vi "ACR_APXStand170322.vi"() -> ()   [LabVIEW 2015]
uses:
  <vilib>/Platform/TimedLoop/XDataNode/timing_clust.ctl
  <vilib>/Platform/TimedLoop/XDataNode/nitl_modes.ctl
  <vilib>/Platform/TimedLoop/XDataNode/wakeup.ctl
  <vilib>/Utility/config.llb/Read Key (String).vi
  <userlib>/caLab/Private/Put_DBL-1D_PV-1D.vi
  <vilib>/platform/TimedLoop/XDataNode/XDataNode.xnode
  <vilib>/Platform/TimedLoop/XDataNode/XDNodeRunTimeDep.lvlib
  <vilib>/Utility/config.llb/NI_LVConfig.lvlib
panel:
  out "COM PORT":i32
  in  "AXIS1 spr":bool
  in  "AXIS4 inc":dbl=0.005 min=0.0 max=0.05 step=0.005 format="%.3f"
  in  "AXIS4 spr":bool
  in  "AXIS4 srl":bool
  out "APX:AXIS4_INSPR":dbl
  in  "AXIS2 spr":bool
  in  "AXIS2 srl":bool
  in  "AXIS2 inc":dbl=0.005 min=0.0 max=0.05 step=0.005 format="%.3f"
  out "APX:AXIS2_TRAN":dbl
  in  "AXIS1 srl":bool
  in  "AXIS1 inc":dbl=0.005 min=0.0 max=0.2 step=0.005 format="%.3f"
  out "APX:AXIS1_INSRL":dbl
  in  "APX:AXIS5_ENB":bool
  in  "APX:AXIS4_ENB":bool
  in  "APX:AXIS3_ENB":bool
  in  "APX:AXIS2_ENB":bool
  in  "APX:AXIS1_ENB":bool
  in  "APX:AXIS0_ENB":bool
  out "error out":errorcluster
  out "APX:AXIS5_ENB":bool
  out "APX:AXIS2_EBD":bool
  out "APX:AXIS1_EBD":bool
  out "APX:AXIS3EBD":bool
  out "APX:AXIS4_EBD":bool
  out "APX:AXIS0_EBD":bool
  out "EPICS error out":errorcluster
  out "ACR error out":errorcluster
  in  "stop":bool
  in  "Write String PROG1":string[](array[string])=["detach all", "new all", "clear", "attach master0", "attach slave0 axis0 \"x\"", "axis0 drive on"]
  in  "AXIS5 down":bool
  in  "AXIS5 up":bool
  in  "AXIS5 inc":dbl=0.01 min=0.0 max=0.2 step=0.005 format="%#.6f"
  in  "AXIS3 down":bool
  in  "AXIS3 up":bool
  in  "AXIS3 inc":dbl=0.005 min=0.0 max=0.2 step=0.005 format="%.3f"
  out "APX:AXIS3_SPRSRL":dbl
  in  "AXIS0 inc":dbl=0.005 min=0.0 max=0.2 step=0.005 format="%.3f"
  in  "AXIS0 down":bool
  in  "AXIS0 up":bool
  out "APX:AXIS5_SPRSRL_ACC":dbl
  out "APX:AXIS4_INSPR_ACC":dbl
  out "APX:AXIS3_SPRSRL_ACC":dbl
  out "APX:AXIS2_TRAN_ACC":dbl
  out "APX:AXIS1_INSRL_ACC":dbl
  out "APX:AXIS0 ZSRL_ACC":dbl
  out "APX:AXIS5_SPRSRL_VEL":dbl
  out "APX:AXIS4_INSPR_VEL":dbl
  out "APX:AXIS3_SPRSRL_VEL":dbl
  out "APX:AXIS2_TRAN_VEL":dbl
  out "APX:AXIS1_INSRL_VEL":dbl
  out "APX:AXIS0_ZSRL_VEL":dbl
  out "APX:AXIS5_SPRSRL":dbl
  in  "nPort":i32=28
  in  "Sampling Time (s)":dbl=0.2
  out "APX:AXIS0_ZSRL":dbl
  in  "Read error in \n(no error)":errorcluster
  in  "Move CMD":string="x/100"
  in  "OK Button":bool
  in  "Write String PROG0":string[](array[string])=["detach all", "new all", "clear", "attach master0", "attach slave0 axis0 \"x\"", "axis0 drive on"]
  out "Terminal Status":bool
  in  "ComACRServerLib.IChannel":refnum<k7>
  in  "bstrIP Property":string="192.168.10.40"
  out "Connect error out":errorcluster
  in  "Connect error in \n(no error)":errorcluster
  # "Ethernet Configuration"
  # "Command"
  # "Configure"
  # "APX\nACR9000 USB"
  # "detach all\nnew all\nclear\nattach master0\nattach slave0 axis0 \"x\"\naxis0 drive on"
  # "Position"
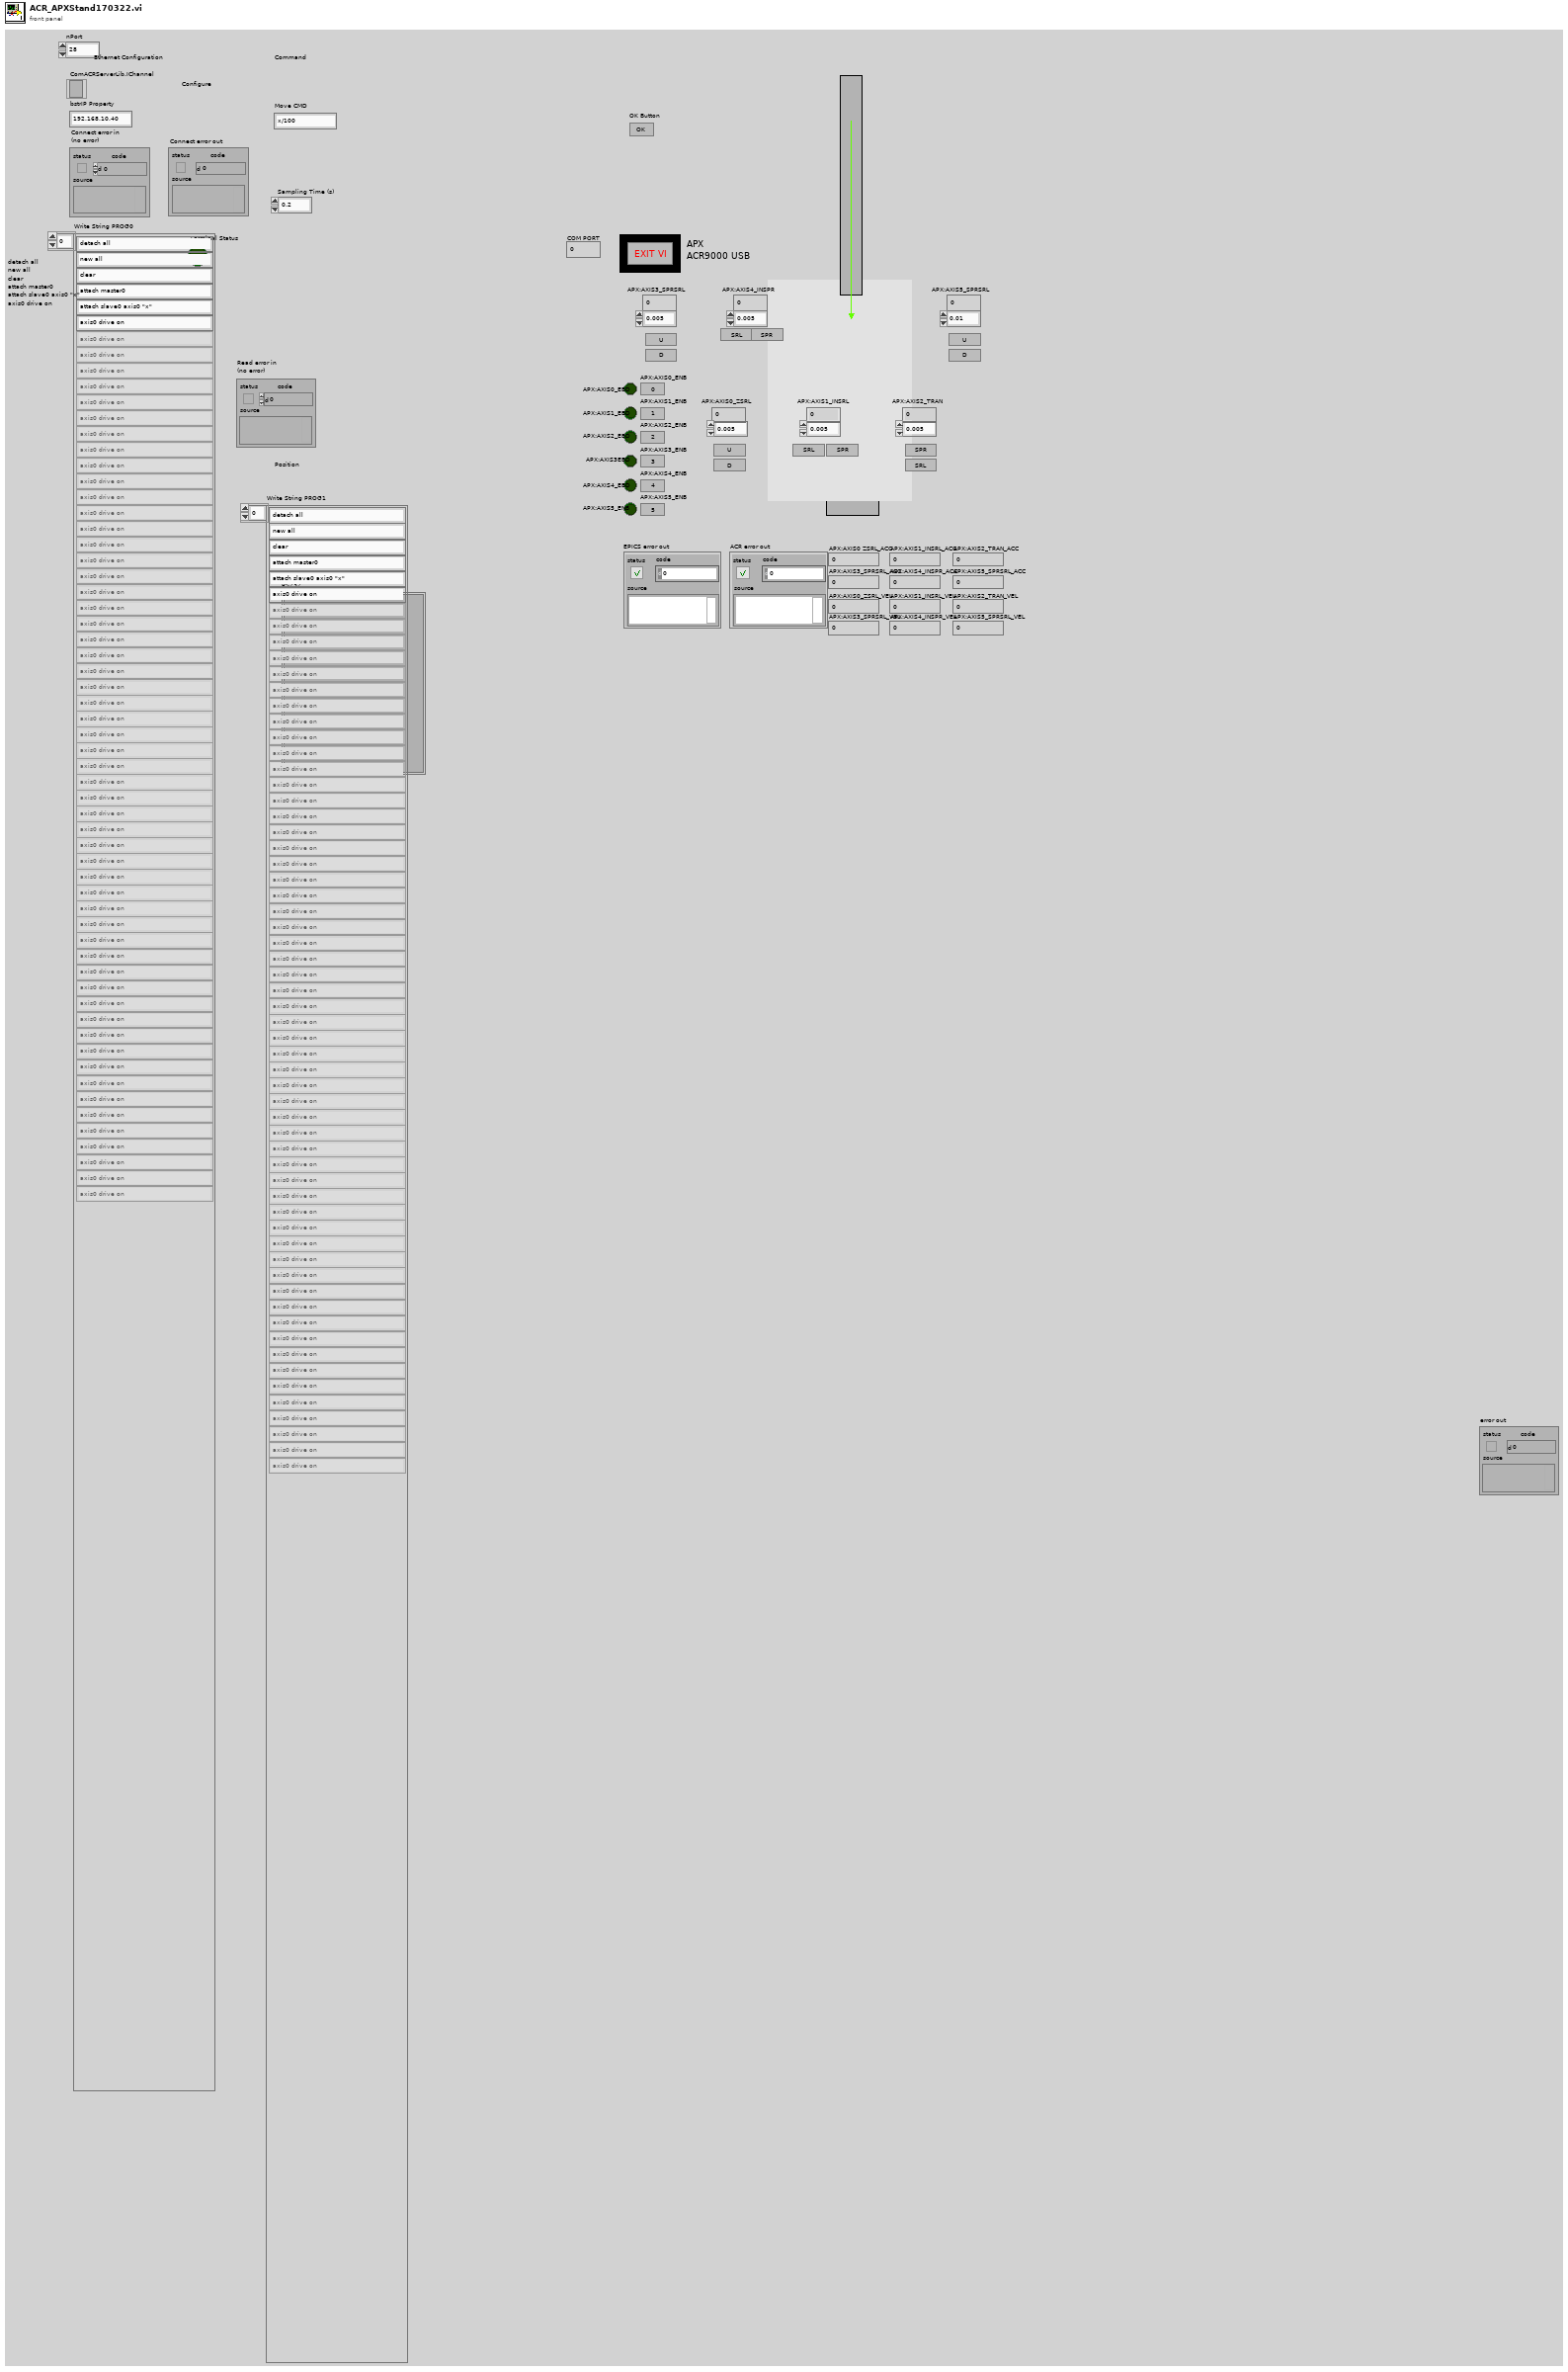
[diagram p1: front panel]
types:
  T1 = typedef "NI_LVConfig.lvlib/Config Data RefNum.ctl" = refnum<k1>
  T2 = typedef "XDNodeRunTimeDep.lvlib/timing_clust.ctl" = cluster{"Expected End [f-1]":u64, "Actual End [f-1]":u64, "Finished Late? [f-1]":bool, "Expected End [i-1]":u64, "Actual End [i-1]":u64, "Finished Late? [i-1]":bool, "Expected Start [i]":u64, "Actual Start [i]":u64, "Expected Start [f]":u64, "Actual Start [f]":u64, "Source Name":string, "Structure Name":string, "Period":i64, "Deadline":i64, "Offset":i64, "Start":i64, "Priority":i32, "Timeout":i32, "Mode":T3, "Wakeup Reason":T4, "Error":errorcluster, "Source Type":string, "Secondary Source Type":string, "Global End Time":u64, "Global Start Time":u64, "Frame Duration":u64, "Iteration Duration":u64, "Assigned CPU":i32, "I/O Scan Engine Mode":u32}
  T3 = typedef "XDNodeRunTimeDep.lvlib/nitl_modes.ctl" = enum32{"No Change", "Process missed periods, maintain original phase", "Discard missed periods, maintain original phase", "Process missed periods, ignore original phase", "Discard missed periods, ignore original phase"}
  T4 = typedef "XDNodeRunTimeDep.lvlib/wakeup.ctl" = enum32{"Normal", "Aborted", "Asynchronous wakeup", "Timing source error", "Timed loop error", "Timeout"}
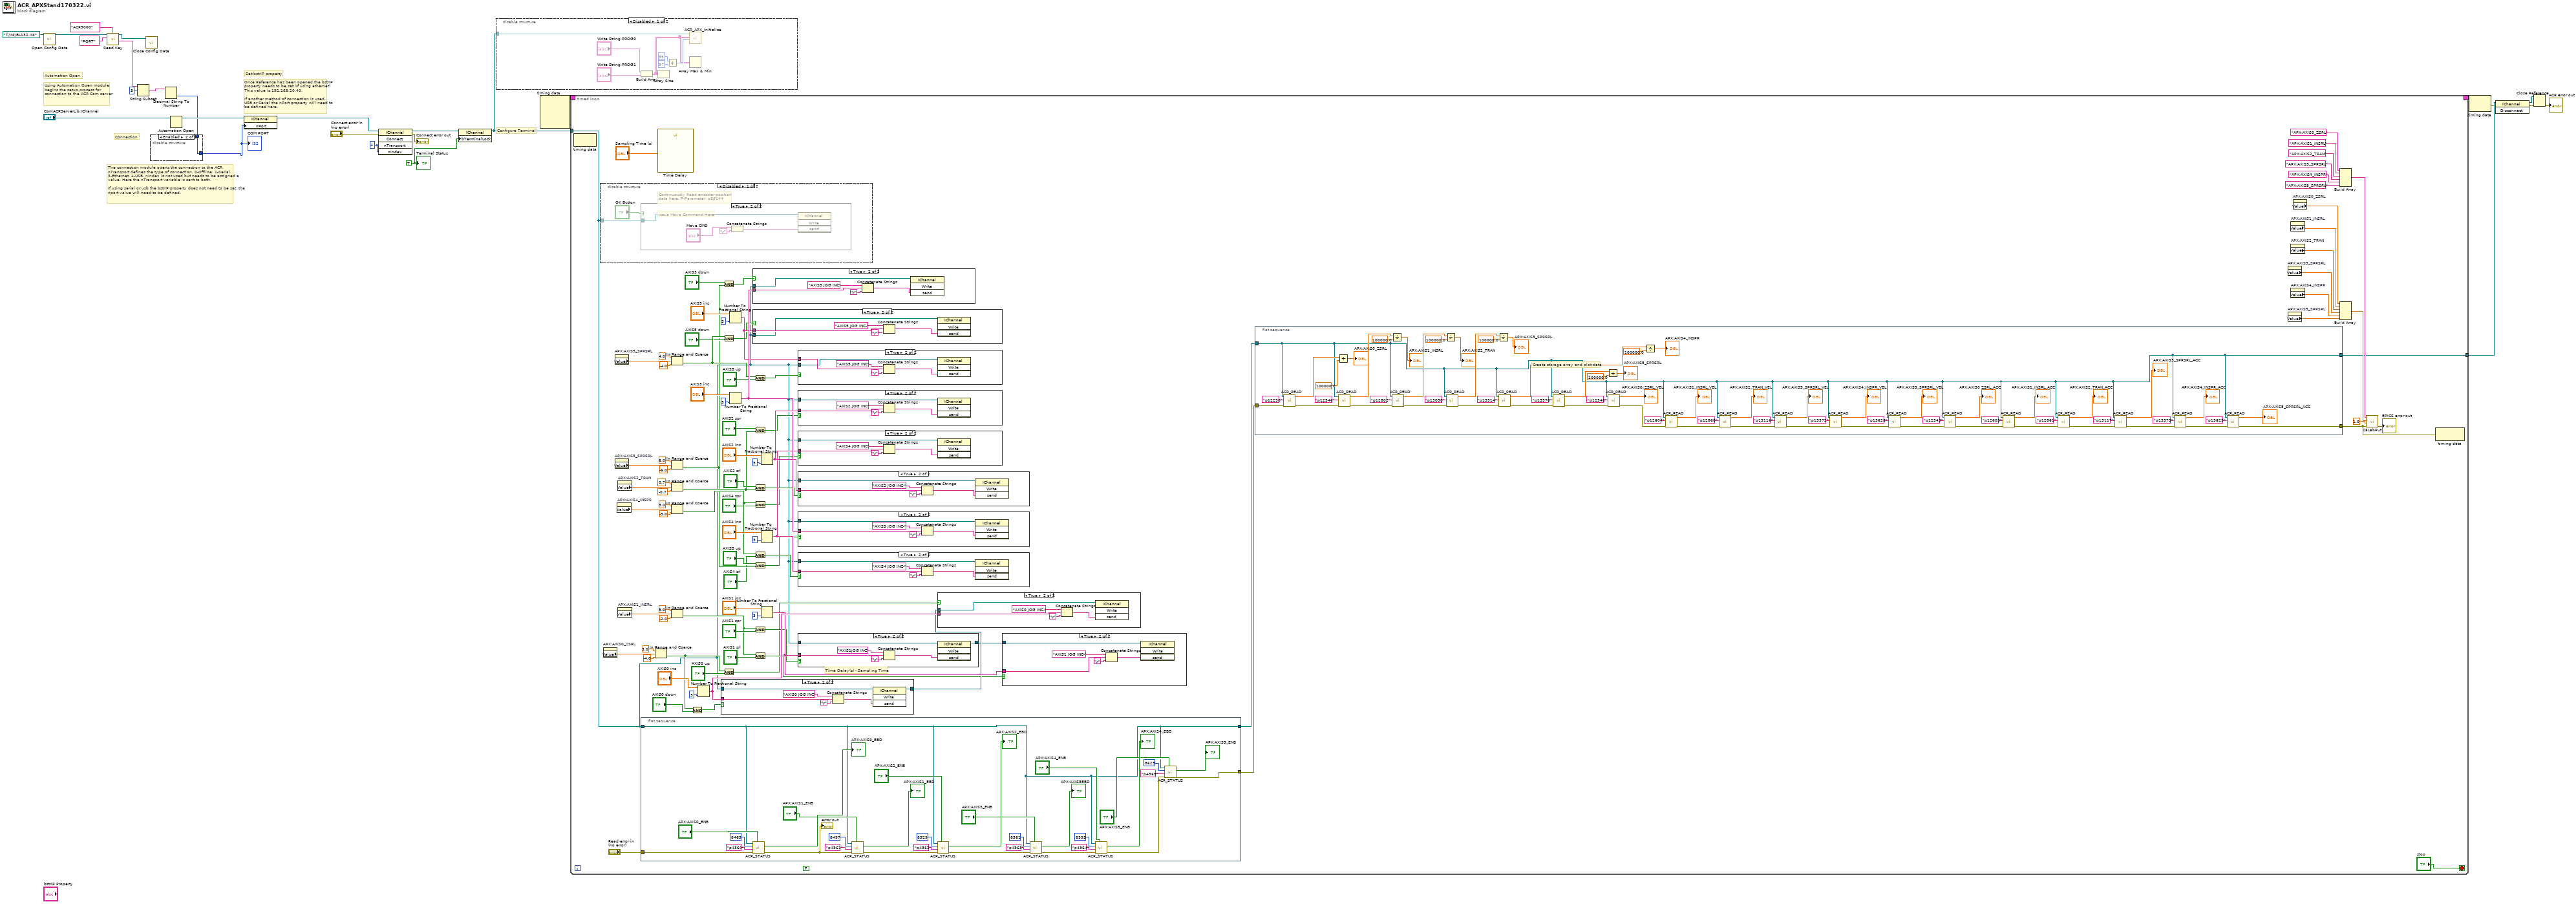
[diagram p0: block diagram]
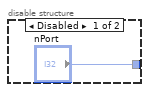
[diagram p2: hidden frame]
diagram:
  w19 = TRUE
  w23 = 4
  # "Configure Terminal"
  # "Using Automation Open module begins the setup process for connection to the ACR Com server"
  # "Automation Open"
  # "Once Reference has been opened,the bstrIP property needs to be set.(If using ethernet) This value is 192.168.10.40. \n\nIf another method of connection is used, USB or Serial the nPort property will need to be defined here."
  # "Set bstrIP property"
  # "The connection module opens the connection to the ACR. nTransport defines the type of connection. 0-Offline, 2-Serial, 3-Ethernet, 4-USB. nIndex is not used but needs to be assigned a value. Here the nTransport variable is sent to both.\n\nIf using serial or usb the bstrIP property does not need to be set; the nport value will need to be defined."
  # "Connection"
  n1 = call <vilib>:"Open Config Data.vi"("configuration file path"=path "T:/INI/BL132.INI") -> ("refnum"=w7:T1)  [unwired: 8 in, 2 out]
  n2 = call-poly <vilib>:"Read Key.vi"("section"="ACR9000" ("y"), "key"="PORT" ("y"), "refnum"=w7) -> ("value"=w5:string, "refnum out"=w6:T1)  [unwired: 5 in, 2 out]
  n3 = String Subset(string=w5, offset (0)=3) -> (substring=w3:string)  [unwired: 1 in]
  n4 = call <vilib>:"Close Config Data.vi"("refnum"=w6) -> ()  [unwired: 9 in, 2 out]
  n5 = Decimal String To Number(string=w3) -> (number=w1:i32)  [unwired: 2 in, 1 out]
  n6 = disable-structure shown="Enabled" {
    disable-tunnel: ["nPort" w28] -> w2
    disable-tunnel: w1 -> [_ w28]
    frame Disabled {
    }
    frame Enabled {
    }
  }
  "COM PORT" <- w2
  n7 = Automation Open(Automation Refnum="ComACRServerLib.IChannel") -> (Automation Refnum=w22:refnum<k7>)  [unwired: 1 in, 3 out]
  n8 = property class="IChannel"(reference=w22, "nPort"=w2) -> (reference out=w21:refnum<k7>)  [unwired: 1 in, 1 out]
  n9 = invoke class="IChannel" method="Connect"(reference=w21, error in="Connect error in \n(no error)", "nTransport"=w23, "nIndex"=w23) -> (reference out=w20:refnum<k7>, error out=→"Connect error out":errorcluster)  [unwired: 1 in, 3 out]
  n10 = property class="IChannel"(reference=w20, "bTerminalLock"=w19) -> (reference out=w18:refnum<k7>)  [unwired: 1 in, 1 out]
  n11 = disable-structure shown="Disabled" {
    disable-tunnel: w18 -> [w35 _]
    frame Disabled {
      n12 = Build Array("Write String PROG0", "Write String PROG1") -> (w29:string[][])
      n13 = Array Size(array=w29) -> ()  [unwired: 1 out]
      n14 = Add(x=99, y=97) -> (x+y=w32:i32)
      n15 = call "ACR_APX_Initialize.vi"("Numeric"=w32, "Array"=w29, "Automation Refnum in"=w35) -> ()  [unwired: 9 in]
      n16 = Array Max & Min(array=w29) -> ()  [unwired: 4 out]
    }
    frame Enabled {
    }
  }
  n17 = node-c288() -> (w17:T2)  [unwired: 4 in]
  n18 = timed-loop {
    tunnel: w18 -> [w40]
    timing: w17 -> [_]
    timing-out: [_] -> w16
    tunnel: [w36] -> w13
    stop <- "stop" stop-if-true
    (unwired) FALSE
    # "Time Delay(s) - Sampling Time"
    n19 = node-c288() -> ()  [unwired: 1 in, 1 out]
    n20 = disable-structure shown="Disabled" {
      disable-tunnel: w40 -> [w228 _]
      frame Disabled {
        # "Continuously Read encoder position\ndata here. P-Parameter: p38144"
        n21 = case shown="True" "OK Button" {
          tunnel: w228 -> [_ w230]
          frame False {
          }
          frame True {
            # "Issue Move Command Here"
            n22 = Concatenate Strings("Move CMD", "\r") -> (w233:string)
            n23 = invoke class="IChannel" method="Write"(reference=w230, "send"=w233) -> ()  [unwired: 2 in, 4 out]
          }
        }
      }
      frame Enabled {
      }
    }
    n24 = property on="APX:AXIS0_ZSRL" class="DigNum (strict)"() -> ("Value"=w48:dbl)  [unwired: 2 in, 2 out]
    n25 = property on="APX:AXIS5_SPRSRL" class="DigNum (strict)"() -> ("Value"=w90:dbl)  [unwired: 2 in, 2 out]
    n26 = property on="APX:AXIS3_SPRSRL" class="DigNum (strict)"() -> ("Value"=w74:dbl)  [unwired: 2 in, 2 out]
    n27 = property on="APX:AXIS4_INSPR" class="DigNum (strict)"() -> ("Value"=w66:dbl)  [unwired: 2 in, 2 out]
    n28 = property on="APX:AXIS2_TRAN" class="DigNum (strict)"() -> ("Value"=w82:dbl)  [unwired: 2 in, 2 out]
    n29 = property on="APX:AXIS1_INSRL" class="DigNum (strict)"() -> ("Value"=w56:dbl)  [unwired: 2 in, 2 out]
    n30 = flat-sequence {
      tunnel: "Read error in \n(no error)" -> [w227]
      tunnel: [w196] -> w37
      tunnel: w40 -> [w196]
      tunnel: [w198] -> w38
      frame #0 {
        n31 = call "ACR_STATUS.vi"("EnableDrive"="APX:AXIS0_ENB", "error in (no error)"=w227, "bstrRequest"="p4360", "nBit"=8465, "Automation Refnum in"=w196) -> ("error out"=w222:errorcluster, "DrvEnaOut"=→"APX:AXIS0_EBD":bool)  [unwired: 4 in, 1 out]
        "error out" <- w222
        n32 = call "ACR_STATUS.vi"("EnableDrive"="APX:AXIS1_ENB", "error in (no error)"=w222, "bstrRequest"="p4361", "nBit"=8497, "Automation Refnum in"=w196) -> ("error out"=w217:errorcluster, "DrvEnaOut"=→"APX:AXIS1_EBD":bool)  [unwired: 4 in, 1 out]
        n33 = call "ACR_STATUS.vi"("EnableDrive"="APX:AXIS2_ENB", "error in (no error)"=w217, "bstrRequest"="p4362", "nBit"=8529, "Automation Refnum in"=w196) -> ("error out"=w212:errorcluster, "DrvEnaOut"=→"APX:AXIS2_EBD":bool)  [unwired: 4 in, 1 out]
        n34 = call "ACR_STATUS.vi"("EnableDrive"="APX:AXIS3_ENB", "error in (no error)"=w212, "bstrRequest"="p4363", "nBit"=8561, "Automation Refnum in"=w196) -> ("error out"=w207:errorcluster, "DrvEnaOut"=→"APX:AXIS3EBD":bool)  [unwired: 4 in, 1 out]
        n35 = call "ACR_STATUS.vi"("EnableDrive"="APX:AXIS4_ENB", "error in (no error)"=w207, "bstrRequest"="p4364", "nBit"=8593, "Automation Refnum in"=w196) -> ("error out"=w202:errorcluster, "DrvEnaOut"=→"APX:AXIS4_EBD":bool)  [unwired: 4 in, 1 out]
        n36 = call "ACR_STATUS.vi"("EnableDrive"="APX:AXIS5_ENB", "error in (no error)"=w202, "bstrRequest"="p4365", "nBit"=8625, "Automation Refnum in"=w196) -> ("error out"=w198:errorcluster, "DrvEnaOut"=→"APX:AXIS5_ENB":bool)  [unwired: 4 in, 1 out]
      }
    }
    n37 = In Range and Coerce(upper limit=5.0, x=w48, lower limit=-4.0) -> (In Range?=w43:bool)  [unwired: 1 out]
    n38 = call "Time Delay"("Delay Time (s)"="Sampling Time (s)") -> ()  [unwired: 1 in, 10 out]
    n39 = In Range and Coerce(upper limit=4.0, x=w90, lower limit=-4.0) -> (In Range?=w85:bool)  [unwired: 1 out]
    n40 = In Range and Coerce(upper limit=6.0, x=w74, lower limit=-6.0) -> (In Range?=w71:bool)  [unwired: 1 out]
    n41 = In Range and Coerce(upper limit=0.7, x=w82, lower limit=-0.7) -> (In Range?=w79:bool)  [unwired: 1 out]
    n42 = In Range and Coerce(upper limit=3.0, x=w66, lower limit=-3.0) -> (In Range?=w64:bool)  [unwired: 1 out]
    n43 = In Range and Coerce(upper limit=3.0, x=w56, lower limit=-2.0) -> (In Range?=w51:bool)  [unwired: 1 out]
    n44 = And(x=w43, y="AXIS0 down") -> (x .and. y?=w46:bool)
    n45 = Number To Fractional String(number="AXIS0 inc", precision (6)=i16 3) -> (F-format string=w124:string)  [unwired: 2 in]
    n46 = case shown="True" w46 {
      tunnel: w124 -> [_ w295]
      tunnel: w40 -> [w290 w292]
      tunnel: [w290 w291] -> w108
      frame False {
      }
      frame True {
        n47 = Concatenate Strings("AXIS0 JOG INC", w295, "\r") -> (w293:string)
        n48 = invoke class="IChannel" method="Write"(reference=w292, "send"=w293) -> (reference out=w291:refnum<k7>)  [unwired: 2 in, 3 out]
      }
    }
    n49 = And(x="AXIS3 down", y=w71) -> (x .and. y?=w68:bool)
    n50 = And(x=w85, y="AXIS5 down") -> (x .and. y?=w83:bool)
    n51 = And(x=w43, y="AXIS0 up") -> (x .and. y?=w44:bool)
    n52 = Number To Fractional String(number="AXIS5 inc", precision (6)=i16 3) -> (F-format string=w110:string)  [unwired: 2 in]
    n53 = Number To Fractional String(number="AXIS3 inc", precision (6)=i16 3) -> (F-format string=w116:string)  [unwired: 2 in]
    n54 = case shown="True" w68 {
      tunnel: w116 -> [_ w261]
      tunnel: w40 -> [_ w258]
      frame False {
      }
      frame True {
        n55 = Concatenate Strings("AXIS3 JOG INC", w261, "\r") -> (w259:string)
        n56 = invoke class="IChannel" method="Write"(reference=w258, "send"=w259) -> ()  [unwired: 2 in, 4 out]
      }
    }
    n57 = case shown="True" w83 {
      tunnel: w110 -> [_ w246]
      tunnel: w40 -> [_ w243]
      frame False {
      }
      frame True {
        n58 = Concatenate Strings("AXIS5 JOG INC-", w246, "\r") -> (w244:string)
        n59 = invoke class="IChannel" method="Write"(reference=w243, "send"=w244) -> ()  [unwired: 2 in, 4 out]
      }
    }
    n60 = And(x=w85, y="AXIS5 up") -> (x .and. y?=w86:bool)
    n61 = And(x="AXIS2 spr", y=w79) -> (x .and. y?=w75:bool)
    n62 = And(x="AXIS2 srl", y=w79) -> (x .and. y?=w77:bool)
    n63 = And(x=w64, y="AXIS4 spr") -> (x .and. y?=w62:bool)
    n64 = And(x=w64, y="AXIS4 srl") -> (x .and. y?=w60:bool)
    n65 = And(x="AXIS3 up", y=w71) -> (x .and. y?=w67:bool)
    n66 = And(x=w51, y="AXIS1 spr") -> (x .and. y?=w52:bool)
    n67 = And(x=w51, y="AXIS1 srl") -> (x .and. y?=w54:bool)
    n68 = Number To Fractional String(number="AXIS2 inc", precision (6)=i16 3) -> (F-format string=w119:string)  [unwired: 2 in]
    n69 = Number To Fractional String(number="AXIS4 inc", precision (6)=i16 3) -> (F-format string=w113:string)  [unwired: 2 in]
    n70 = Number To Fractional String(number="AXIS1 inc", precision (6)=i16 3) -> (F-format string=w122:string)  [unwired: 2 in]
    n71 = case shown="True" w86 {
      tunnel: w110 -> [_ w241]
      tunnel: w40 -> [_ w238]
      frame False {
      }
      frame True {
        n72 = Concatenate Strings("AXIS5 JOG INC", w241, "\r") -> (w239:string)
        n73 = invoke class="IChannel" method="Write"(reference=w238, "send"=w239) -> ()  [unwired: 2 in, 4 out]
      }
    }
    n74 = case shown="True" w75 {
      tunnel: w119 -> [_ w271]
      tunnel: w40 -> [_ w268]
      frame False {
      }
      frame True {
        n75 = Concatenate Strings("AXIS2 JOG INC", w271, "\r") -> (w269:string)
        n76 = invoke class="IChannel" method="Write"(reference=w268, "send"=w269) -> ()  [unwired: 2 in, 4 out]
      }
    }
    n77 = case shown="True" w62 {
      tunnel: w113 -> [_ w251]
      tunnel: w40 -> [_ w248]
      frame False {
      }
      frame True {
        n78 = Concatenate Strings("AXIS4 JOG INC", w251, "\r") -> (w249:string)
        n79 = invoke class="IChannel" method="Write"(reference=w248, "send"=w249) -> ()  [unwired: 2 in, 4 out]
      }
    }
    n80 = case shown="True" w77 {
      tunnel: w119 -> [_ w276]
      tunnel: w40 -> [_ w274]
      frame False {
      }
      frame True {
        n81 = Concatenate Strings("AXIS2 JOG INC-", w276, "\r") -> (w273:string)
        n82 = invoke class="IChannel" method="Write"(reference=w274, "send"=w273) -> ()  [unwired: 2 in, 4 out]
      }
    }
    n83 = case shown="True" w67 {
      tunnel: w116 -> [_ w266]
      tunnel: w40 -> [_ w263]
      frame False {
      }
      frame True {
        n84 = Concatenate Strings("AXIS3 JOG INC-", w266, "\r") -> (w264:string)
        n85 = invoke class="IChannel" method="Write"(reference=w263, "send"=w264) -> ()  [unwired: 2 in, 4 out]
      }
    }
    n86 = case shown="True" w60 {
      tunnel: w113 -> [_ w256]
      tunnel: w40 -> [_ w253]
      frame False {
      }
      frame True {
        n87 = Concatenate Strings("AXIS4 JOG INC-", w256, "\r") -> (w254:string)
        n88 = invoke class="IChannel" method="Write"(reference=w253, "send"=w254) -> ()  [unwired: 2 in, 4 out]
      }
    }
    n89 = case shown="True" w52 {
      tunnel: w122 -> [_ w283]
      tunnel: w40 -> [w278 w280]
      tunnel: [w278 w279] -> w107
      frame False {
      }
      frame True {
        n90 = Concatenate Strings("AXIS1JOG INC", w283, "\r") -> (w281:string)
        n91 = invoke class="IChannel" method="Write"(reference=w280, "send"=w281) -> (reference out=w279:refnum<k7>)  [unwired: 2 in, 3 out]
      }
    }
    n92 = case shown="True" w44 {
      tunnel: w124 -> [_ w300]
      tunnel: w108 -> [_ w297]
      frame False {
      }
      frame True {
        n93 = Concatenate Strings("AXIS0 JOG INC-", w300, "\r") -> (w298:string)
        n94 = invoke class="IChannel" method="Write"(reference=w297, "send"=w298) -> ()  [unwired: 2 in, 4 out]
      }
    }
    n95 = case shown="True" w54 {
      tunnel: w122 -> [_ w288]
      tunnel: w107 -> [_ w285]
      frame False {
      }
      frame True {
        n96 = Concatenate Strings("AXIS1 JOG INC-", w288, "\r") -> (w286:string)
        n97 = invoke class="IChannel" method="Write"(reference=w285, "send"=w286) -> ()  [unwired: 2 in, 4 out]
      }
    }
    n98 = flat-sequence {
      tunnel: [w130] -> w42
      tunnel: w38 -> [w129]
      tunnel: w37 -> [w128]
      tunnel: [w128] -> w36
      frame #0 {
        # "Create storage array and plot data"
        n99 = call "ACR_READ.vi"("error in (no error)"=w129, "Actual"="p12290", "Automation Refnum in"=w128) -> ("error out"=w194:errorcluster, "AXIS0"=w147:dbl)  [unwired: 7 in]
        n100 = Divide(x=w147, y=100000.0) -> (x/y=→"APX:AXIS0_ZSRL":dbl)
        n101 = call "ACR_READ.vi"("error in (no error)"=w194, "Actual"="p12546", "Automation Refnum in"=w128) -> ("error out"=w193:errorcluster, "AXIS0"=w144:dbl)  [unwired: 7 in]
        n102 = Divide(x=w144, y=100000.0) -> (x/y=→"APX:AXIS1_INSRL":dbl)
        n103 = call "ACR_READ.vi"("error in (no error)"=w193, "Actual"="p12802", "Automation Refnum in"=w128) -> ("error out"=w192:errorcluster, "AXIS0"=w141:dbl)  [unwired: 7 in]
        n104 = Divide(x=w141, y=100000.0) -> (x/y=→"APX:AXIS2_TRAN":dbl)
        n105 = call "ACR_READ.vi"("error in (no error)"=w192, "Actual"="p13058", "Automation Refnum in"=w128) -> ("error out"=w191:errorcluster, "AXIS0"=w138:dbl)  [unwired: 7 in]
        n106 = Divide(x=w138, y=100000.0) -> (x/y=→"APX:AXIS3_SPRSRL":dbl)
        n107 = call "ACR_READ.vi"("error in (no error)"=w191, "Actual"="p13314", "Automation Refnum in"=w128) -> ("error out"=w190:errorcluster, "AXIS0"=w135:dbl)  [unwired: 7 in]
        n108 = call "ACR_READ.vi"("error in (no error)"=w190, "Actual"="p13570", "Automation Refnum in"=w128) -> ("error out"=w179:errorcluster, "AXIS0"=w132:dbl)  [unwired: 7 in]
        n109 = Divide(x=w132, y=100000.0) -> (x/y=→"APX:AXIS5_SPRSRL":dbl)
        n110 = call "ACR_READ.vi"("error in (no error)"=w179, "Actual"="p12348", "Automation Refnum in"=w128) -> ("error out"=w184:errorcluster, "AXIS0"=→"APX:AXIS0_ZSRL_VEL":dbl)  [unwired: 7 in]
        n111 = Divide(x=w135, y=100000.0) -> (x/y=→"APX:AXIS4_INSPR":dbl)
        n112 = call "ACR_READ.vi"("error in (no error)"=w184, "Actual"="p12604", "Automation Refnum in"=w128) -> ("error out"=w183:errorcluster, "AXIS0"=→"APX:AXIS1_INSRL_VEL":dbl)  [unwired: 7 in]
        n113 = call "ACR_READ.vi"("error in (no error)"=w183, "Actual"="p12860", "Automation Refnum in"=w128) -> ("error out"=w182:errorcluster, "AXIS0"=→"APX:AXIS2_TRAN_VEL":dbl)  [unwired: 7 in]
        n114 = call "ACR_READ.vi"("error in (no error)"=w182, "Actual"="p13116", "Automation Refnum in"=w128) -> ("error out"=w181:errorcluster, "AXIS0"=→"APX:AXIS3_SPRSRL_VEL":dbl)  [unwired: 7 in]
        n115 = call "ACR_READ.vi"("error in (no error)"=w181, "Actual"="p13372", "Automation Refnum in"=w128) -> ("error out"=w180:errorcluster, "AXIS0"=→"APX:AXIS4_INSPR_VEL":dbl)  [unwired: 7 in]
        n116 = call "ACR_READ.vi"("error in (no error)"=w180, "Actual"="p13628", "Automation Refnum in"=w128) -> ("error out"=w155:errorcluster, "AXIS0"=→"APX:AXIS5_SPRSRL_VEL":dbl)  [unwired: 7 in]
        n117 = call "ACR_READ.vi"("error in (no error)"=w155, "Actual"="p12349", "Automation Refnum in"=w128) -> ("error out"=w166:errorcluster, "AXIS0"=→"APX:AXIS0 ZSRL_ACC":dbl)  [unwired: 7 in]
        n118 = call "ACR_READ.vi"("error in (no error)"=w166, "Actual"="p12605", "Automation Refnum in"=w128) -> ("error out"=w165:errorcluster, "AXIS0"=→"APX:AXIS1_INSRL_ACC":dbl)  [unwired: 7 in]
        n119 = call "ACR_READ.vi"("error in (no error)"=w165, "Actual"="p12861", "Automation Refnum in"=w128) -> ("error out"=w164:errorcluster, "AXIS0"=→"APX:AXIS2_TRAN_ACC":dbl)  [unwired: 7 in]
        n120 = call "ACR_READ.vi"("error in (no error)"=w164, "Actual"="p13117", "Automation Refnum in"=w128) -> ("error out"=w163:errorcluster, "AXIS0"=→"APX:AXIS3_SPRSRL_ACC":dbl)  [unwired: 7 in]
        n121 = call "ACR_READ.vi"("error in (no error)"=w163, "Actual"="p13373", "Automation Refnum in"=w128) -> ("error out"=w162:errorcluster, "AXIS0"=→"APX:AXIS4_INSPR_ACC":dbl)  [unwired: 7 in]
        n122 = call "ACR_READ.vi"("error in (no error)"=w162, "Actual"="p13629", "Automation Refnum in"=w128) -> ("error out"=w130:errorcluster, "AXIS0"=→"APX:AXIS5_SPRSRL_ACC":dbl)  [unwired: 7 in]
      }
    }
    n123 = property on="APX:AXIS3_SPRSRL" class="DigNum (strict)"() -> ("Value"=w95:dbl)  [unwired: 2 in, 2 out]
    n124 = property on="APX:AXIS5_SPRSRL" class="DigNum (strict)"() -> ("Value"=w93:dbl)  [unwired: 2 in, 2 out]
    n125 = property on="APX:AXIS1_INSRL" class="DigNum (strict)"() -> ("Value"=w97:dbl)  [unwired: 2 in, 2 out]
    n126 = property on="APX:AXIS2_TRAN" class="DigNum (strict)"() -> ("Value"=w96:dbl)  [unwired: 2 in, 2 out]
    n127 = property on="APX:AXIS4_INSPR" class="DigNum (strict)"() -> ("Value"=w94:dbl)  [unwired: 2 in, 2 out]
    n128 = property on="APX:AXIS0_ZSRL" class="DigNum (strict)"() -> ("Value"=w98:dbl)  [unwired: 2 in, 2 out]
    n129 = Build Array("APX:AXIS0_ZSRL", "APX:AXIS1_INSRL", "APX:AXIS2_TRAN", "APX:AXIS3_SPRSRL", "APX:AXIS4_INSPR", "APX:AXIS5_SPRSRL") -> (w91:string[])
    n130 = Build Array(w98, w97, w96, w95, w94, w93) -> (w92:dbl[])
    n131 = call-poly <userlib>:"CaLabPut.vi"("Error in (no error)"=w42, "Timeout (3)"=1.0, "Values"=w92, "PV Names"=w91) -> ("Error out"=→"EPICS error out":errorcluster)  [unwired: 4 in, 3 out]
    n132 = node-c288(w42) -> ()  [unwired: 1 out]
  }
  n133 = node-c288(w16) -> (w11:errorcluster)
  n134 = invoke class="IChannel" method="Disconnect"(reference=w13, error in=w11) -> (reference out=w15:refnum<k7>, error out=w14:errorcluster)  [unwired: 1 in, 1 out]
  n135 = Close Reference(reference=w15, error in (no error)=w14) -> (error out=→"ACR error out":errorcluster)
  "Terminal Status" <- w19
